vi "QueueEnqueueWithPayload.vi"(2 "error in (no error)":errorcluster, 3 "Payload":variant, 4 "Action":T1, 5 "Queue in":refnum<queue>) -> (0 "error out":errorcluster, 1 "Queue out":refnum<queue>)   [LabVIEW 2017]
uses:
  Action.ctl
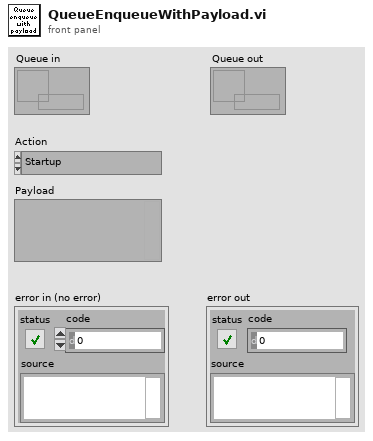
[diagram p1: front panel]
types:
  T1 = typedef "Action.ctl" = enum16{"Startup", "Shutdown", "SaveSettings", "LoadSettings", "InitVNA", "CloseVNA", "InitScan", "IncrementScan", "StopScan", "Target=VNA", "Target=Refrigerator", "Acquire", "Graph", "PNA", "ENA", "ADR", "PPMS"}
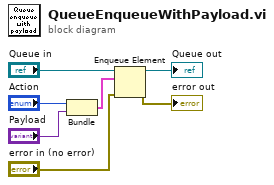
[diagram p0: block diagram]
diagram:
  n1 = Bundle("Action"="Action", "Payload"="Payload") -> (w5:cluster{"Action":T1, "Payload":variant})  [unwired: 1 in]
  n2 = Enqueue Element(queue="Queue in", element=w5, error in (no error)="error in (no error)") -> (queue out=→"Queue out":refnum<queue>, error out=→"error out":errorcluster)  [unwired: 1 in, 1 out]
